vi "Set piezo voltage.vi"(8 "error in (no error)":errorcluster, 10 "Voltage":dbl, 11 "COM port in":refnum<visa-resource-name>) -> (0 "error out":errorcluster, 3 "COM port out":refnum<visa-resource-name>)   [LabVIEW 2020]
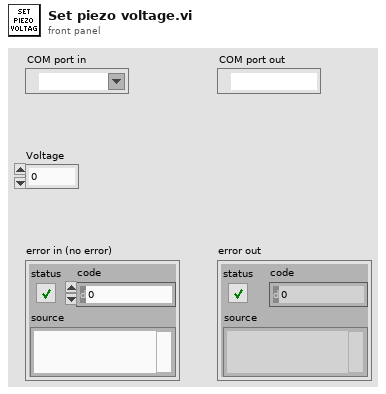
[diagram p1: front panel]
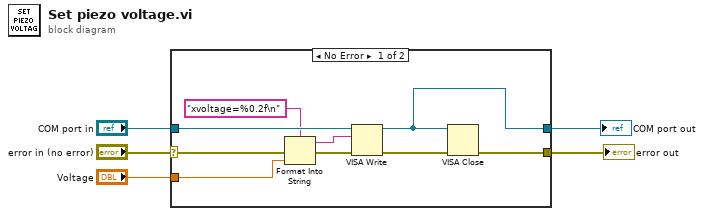
[diagram p0: block diagram]
diagram:
  n1 = case shown="No Error" "error in (no error)" {
    selector: "error in (no error)" -> [w11 w16]
    tunnel: [w7 w16] -> w4
    tunnel: "COM port in" -> [w14 w15]
    tunnel: [w6 w15] -> w2
    tunnel: "Voltage" -> [w9 _]
    frame No Error {
      n2 = Format Into String(format string="xvoltage=%0.2f\n", error in=w11, w9) -> (resulting string=w12:string, error out=w10:errorcluster)  [unwired: 1 in]
      n3 = VISA Write(VISA resource name=w14, write buffer=w12, error in (no error)=w10) -> (VISA resource name out=w6:refnum<visa-resource-name>, error out=w8:errorcluster)  [unwired: 1 out]
      n4 = VISA Close(VISA resource name=w6, error in (no error)=w8) -> (error out=w7:errorcluster)
    }
    frame Error {
    }
  }
  "error out" <- w4
  "COM port out" <- w2
